vi "Read Error.vi"(11 "Iterator Report Error Msg":refnum<class "Iterator Report Error Msg.lvclass">) -> (1 "Stopped by the Caller?":bool, 2 "Error":errorcluster)   [LabVIEW 2017, in "Iterator Actor.lvlib" / "Iterator Report Error Msg.lvclass"]
doc: "Read the Error data and Stopped by the Caller value from the abstract Send Report Error message. \nThis method should be called within the Client Do.vi specified to handle this abstract message."
uses:
  Iterator Report Error Msg.lvclass
  Iterator Report Error Msg.lvclass/Iterator Report Error Msg.ctl
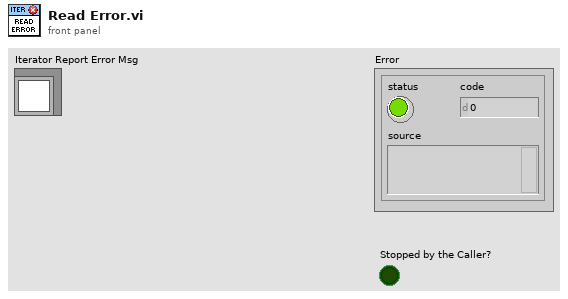
[diagram p1: front panel]
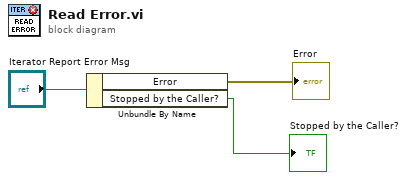
[diagram p0: block diagram]
diagram:
  n1 = Unbundle By Name("Iterator Report Error Msg") -> ("Error"=→"Error":errorcluster, "Stopped by the Caller?"=→"Stopped by the Caller?":bool)
